vi "Get AI Node Value.vi"(10 "Location":i32, 11 "Board State":i32) -> (3 "Value":T1)   [LabVIEW 2013]
uses:
  Typedef/Cell.ctl
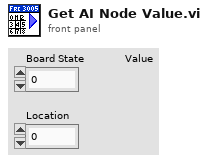
[diagram p1: front panel]
types:
  T1 = typedef "Cell.ctl" = enum16{"", "X", "O"}
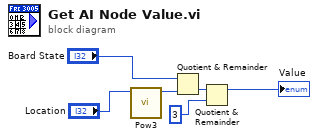
[diagram p0: block diagram]
diagram:
  n1 = call "Pow3.vi"("x"="Location") -> ("x^3"=w4:i32)  [unwired: 10 in]
  n2 = Quotient & Remainder(x="Board State", y=w4) -> (floor(x/y)=w3:i32)  [unwired: 1 out]
  n3 = Quotient & Remainder(x=w3, y=3) -> (x-y*floor(x/y)=→"Value":i32)  [unwired: 1 out]
